vi "Write StartVal.vi"(8 "error in (no error)":errorcluster, 10 "Value":dbl, 11 "TTLController in":refnum<class "TTLController.lvclass">) -> (0 "error out":errorcluster, 3 "TTLController out":refnum<class "TTLController.lvclass">)   [LabVIEW 2020, in "TTLController.lvclass"]
uses:
  TTLController.lvclass
  TTLController.lvclass/TTLController.ctl
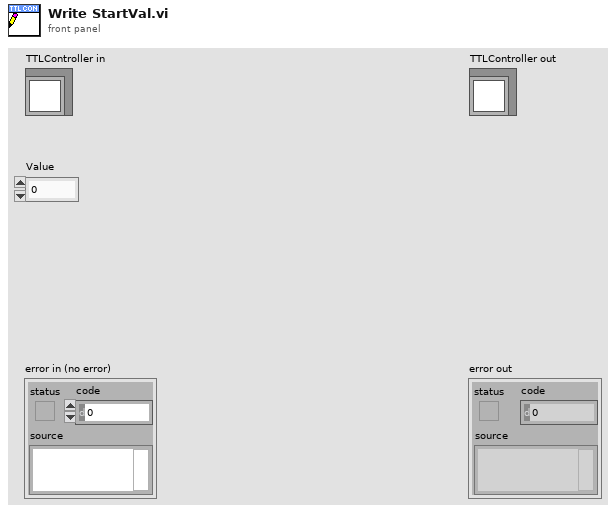
[diagram p1: front panel]
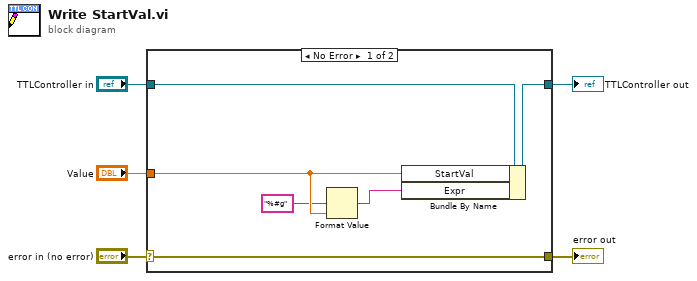
[diagram p0: block diagram]
diagram:
  n1 = case shown="No Error" "error in (no error)" {
    selector: "error in (no error)" -> [w11 w12]
    tunnel: [w11 w12] -> w4
    tunnel: [w9 w13] -> w2
    tunnel: "TTLController in" -> [w10 w13]
    tunnel: "Value" -> [w8 _]
    frame No Error {
      n2 = Format Value(format string="%#g", value (0)=w8) -> (output string=w7:string)  [unwired: 1 in]
      n3 = Bundle By Name(cluster=w10, "StartVal"=w8, "Expr"=w7) -> (w9:refnum<class "TTLController.lvclass">)
    }
    frame Error {
    }
  }
  "error out" <- w4
  "TTLController out" <- w2
